vi "WriteFile.vi"(1 "Enable":bool, 5 "Saving File Path":path, 6 "Alarm":bool, 8 "Length [mm]":dbl, 12 "Speed [m/s]":dbl) -> ()   [LabVIEW 2020]
uses:
  <vilib>/express/express shared/transition.llb/Dynamic To Waveform Array.vi
  <vilib>/express/express signal manip/GetorSetDDTAttributes/Set DDT Attributes/SetT0.vi
  <vilib>/express/express shared/transition.llb/Waveform Array To Dynamic.vi
  <vilib>/express/express signal manip/GetorSetDDTAttributes/Set DDT Attributes/Set DDT Properties.xnode
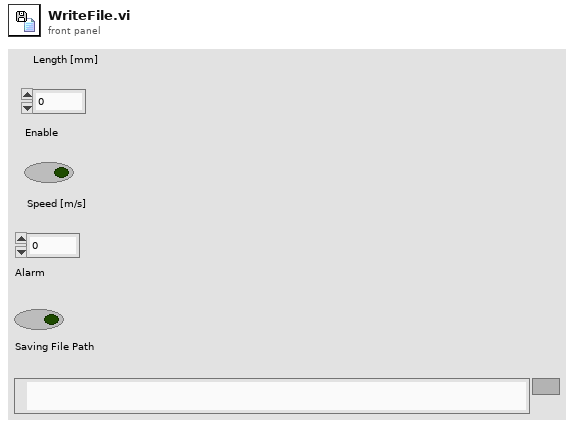
[diagram p1: front panel]
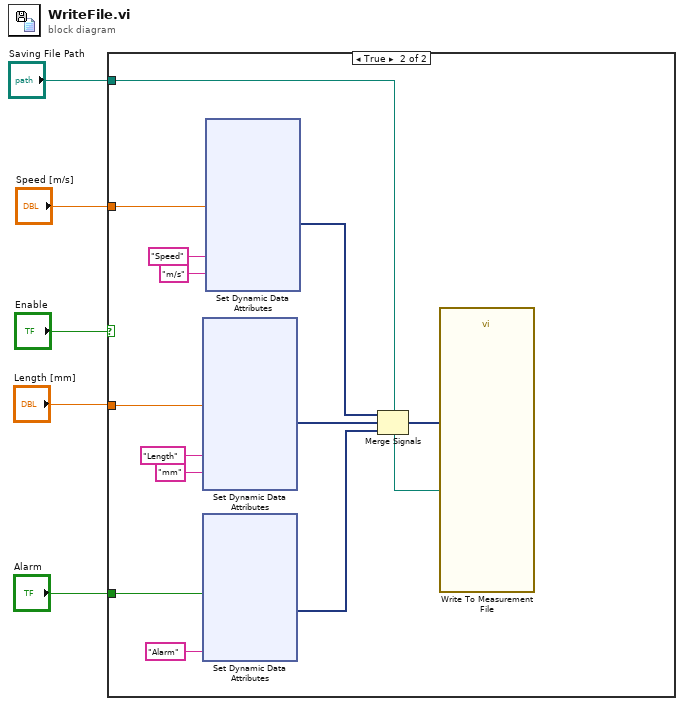
[diagram p0: block diagram]
diagram:
  n1 = case shown="True" "Enable" {
    tunnel: "Speed [m/s]" -> [_ w16]
    tunnel: "Length [mm]" -> [_ w13]
    tunnel: "Alarm" -> [_ w11]
    tunnel: "Saving File Path" -> [_ w6]
    frame False {
    }
    frame True {
      n2 = xnode "Set Dynamic Data Attributes"("Signals In"=w13, "Signal Name"="Length", "Unit"="mm") -> ("Signals Out"=w10:dynamicdata)  [unwired: 2 in, 1 out]
      n3 = xnode "Set Dynamic Data Attributes"("Signals In"=w11, "Signal Name"="Alarm") -> ("Signals Out"=w8:dynamicdata)  [unwired: 2 in, 1 out]
      n4 = xnode "Set Dynamic Data Attributes"("Signals In"=w16, "Signal Name"="Speed", "Unit"="m/s") -> ("Signals Out"=w9:dynamicdata)  [unwired: 2 in, 1 out]
      n5 = Merge Signals(w9, w10, w8) -> (w7:dynamicdata)
      n6 = call "Write To Measurement File"("Signals"=w7, "Filename"=w6) -> ()  [unwired: 15 in, 3 out]
    }
  }
